vi "SubVI_1.vi"(0 "Boolean":bool, 5 "Temp (F)":dbl) -> (4 "Numeric":dbl)   [LabVIEW 2020]
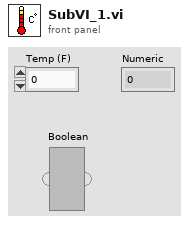
[diagram p1: front panel]
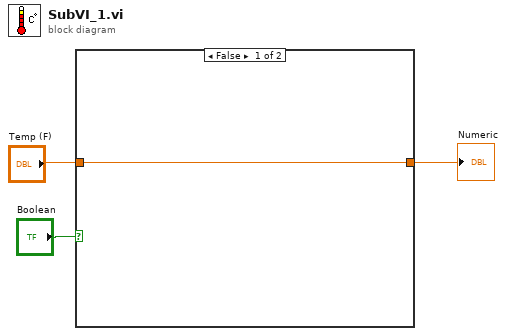
[diagram p0: block diagram]
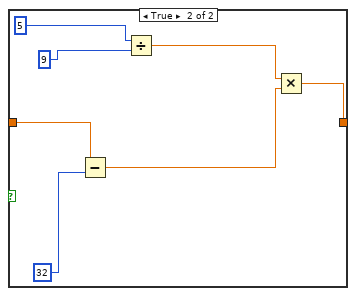
[diagram p2: hidden frame]
diagram:
  n1 = case shown="False" "Boolean" {
    tunnel: "Temp (F)" -> [w4 w11]
    tunnel: [w4 w10] -> w2
    frame False {
    }
    frame True {
      n2 = Subtract(x=w11, y=32) -> (x-y=w6:dbl)
      n3 = Divide(x=5, y=9) -> (x/y=w7:dbl)
      n4 = Multiply(x=w7, y=w6) -> (x*y=w10:dbl)
    }
  }
  "Numeric" <- w2
